vi "Wgrywanie mapy terenu.vi"(11 "Lokalizacja mapy terenu":path) -> (1 "Rectangle":T1, 2 "Mapa terenu":picture)   [LabVIEW 2012, in "Biblioteka moduł map v3.lvlib" / "Obsługa grafiki mapy.lvlib"]
doc: "Zadaniem pliku jest wgranie ze wskazanej lokalizacji wyglądu mapy terenu."
uses:
  <vilib>/picture/picture.llb/imagedata.ctl
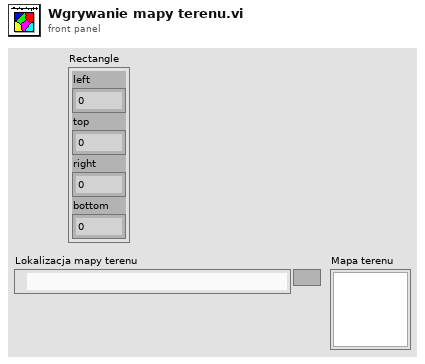
[diagram p1: front panel]
types:
  T1 = cluster{"left":i16, "top":i16, "right":i16, "bottom":i16}
  T2 = typedef "imagedata.ctl" = cluster{"image type":i32, "image depth":i32, "image":u8[], "mask":u8[], "colors":u32[], "Rectangle":cluster{"left":i16, "top":i16, "right":i16, "bottom":i16}}
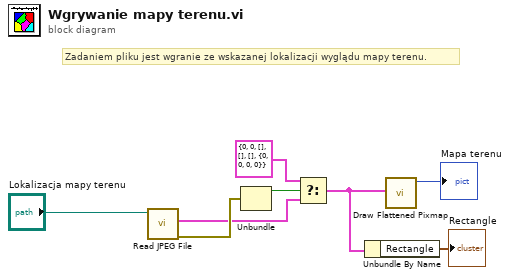
[diagram p0: block diagram]
diagram:
  # "Zadaniem pliku jest wgranie ze wskazanej lokalizacji wyglądu mapy terenu."
  n1 = call <vilib>:"Read JPEG File.vi"("path to JPEG file"="Lokalizacja mapy terenu") -> ("error out"=w6:errorcluster, "image data"=w3:T2)  [unwired: 8 in, 1 out]
  n2 = Unbundle(w6) -> ("status"=w4:bool)  [unwired: 2 out]
  n3 = Select(t=T2 {"image type"=0, "image depth"=0, "image"=[], "mask"=[], "colors"=[], "Rectangle"={"left"=0, "top"=0, "right"=0, "bottom"=0}} ("image data"), s=w4, f=w3) -> (s? t:f=w2:T2)
  n4 = Unbundle By Name(w2) -> ("Rectangle"=→"Rectangle":T1)
  n5 = call <vilib>:"Draw Flattened Pixmap.vi"("image data"=w2) -> ("new picture"=→"Mapa terenu":picture)  [unwired: 8 in]
